vi "Get All Enpoint Configurations.vi"(8 "error in (no error)":errorcluster, 11 "Endpoint Config Section Ref in":T3 format="%.0x") -> (0 "error out":errorcluster, 1 "Endpoints found":bool, 2 "All Endpoint Configurations":T1[](array[typedef]), 3 "Endpoint Config Section Ref out":T3 format="%.0x")   [LabVIEW 2017, in "SLSC Switch Scripting.lvlib"]
uses:
  SLSC Switch Scripting.lvlib
  <vilib>/NI Veristand/Custom Device API/Custom Device Item Ref.ctl
  Endpoint Configuration Cluster.ctl
  Endpoint Configuration Enum.ctl
  <vilib>/NI VeriStand/Custom Device API/Custom Device API.lvlib
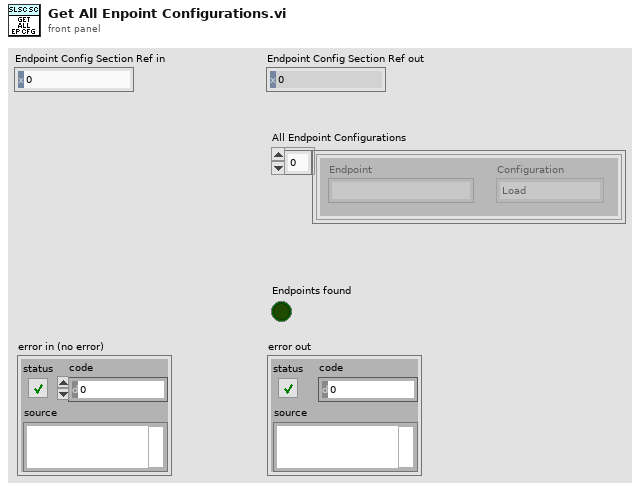
[diagram p1: front panel]
types:
  T1 = typedef "SLSC Switch Scripting.lvlib/Endpoint Configuration Cluster.ctl" = cluster{"Endpoint":string, "Configuration":T2}
  T2 = typedef "SLSC Switch Scripting.lvlib/Endpoint Configuration Enum.ctl" = enum16{"Load", "Source", "Configuration"}
  T3 = typedef "Custom Device API.lvlib/Custom Device Item Ref.ctl" = u64
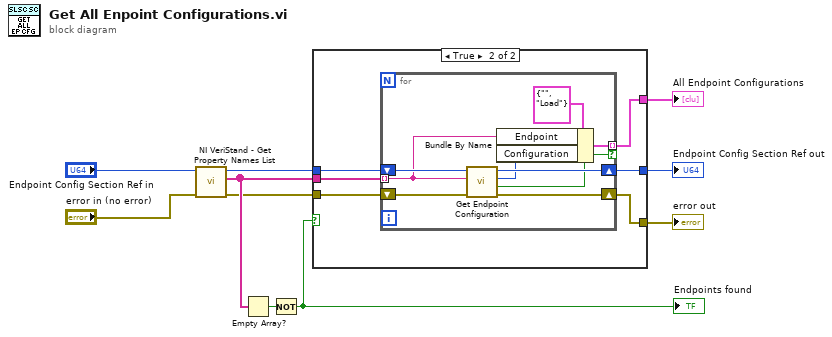
[diagram p0: block diagram]
diagram:
  n1 = call <vilib>:"NI VeriStand - Get Property Names List.vi"("error in (no error)"="error in (no error)", "Item Ref in"="Endpoint Config Section Ref in") -> ("error out"=w8:errorcluster, "Property Names"=w9:string[], "Item Ref out"=w3:T3)  [unwired: 7 in]
  n2 = Empty Array?(array=w9) -> (empty?=w10:bool)
  n3 = Not(x=w10) -> (.not. x?=w1:bool)
  "Endpoints found" <- w1
  n4 = case shown="True" w1 {
    tunnel: w9 -> [_ w18]
    tunnel: w8 -> [w11 w17]
    tunnel: [_ w16] -> w6
    tunnel: [w11 w15] -> w5
    tunnel: w3 -> [w12 w14]
    tunnel: [w12 w13] -> w2
    frame False {
    }
    frame True {
      n5 = for {
        tunnel: w18 -> [w23] mode=indexing
        shift-right: [w21] -> w15
        shift-left: w17 -> [w24]
        tunnel: [w27] -> w16 mode=indexing if=w20
        shift-right: [w25] -> w13
        shift-left: w14 -> [w26]
        n6 = call "Get Endpoint Configuration.vi"("error in (no error)"=w24, "Endpoint"=w23, "Endpoint Config Section Ref in"=w26) -> ("error out"=w21:errorcluster, "Endpoint found"=w20:bool, "Configuration Type"=w22:T2, "Endpoint Config Section Ref out"=w25:T3)  [unwired: 5 in]
        n7 = Bundle By Name(cluster=T1 {"Endpoint"="", "Configuration"=enum."Load"} ("Connection"), "Endpoint"=w23, "Configuration"=w22) -> (w27:T1)
      }
    }
  }
  "error out" <- w5
  "Endpoint Config Section Ref out" <- w2
  "All Endpoint Configurations" <- w6
